vi "power_to_voltage.vi"(11 "Power":dbl) -> (3 "Voltage":dbl)   [LabVIEW 2020]
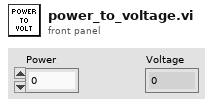
[diagram p1: front panel]
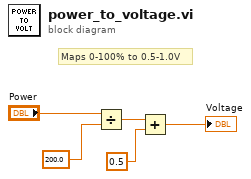
[diagram p0: block diagram]
diagram:
  # "Maps 0-100% to 0.5-1.0V"
  n1 = Divide(x="Power", y=200.0) -> (x/y=w1:dbl)
  n2 = Add(x=w1, y=0.5) -> (x+y=→"Voltage":dbl)
